vi "4Pi Test Astig.vi"(7 "Calling VI Ref":refnum<vi>) -> ()   [LabVIEW 2016]
uses:
  Hardware Configuration/Hardware Configuration Controls/Device Type.ctl
  Hardware Configuration/Hardware Configuration Controls/Device Function.ctl
  <vilib>/Utility/miscctls.llb/LVPointTypeDef.ctl
  4Pi Test Astig - Type Defs/4Pi Test Astig - Actions.ctl
  4Pi Test Astig - Type Defs/4Pi Test Astig - Notifier Type.ctl
  Device Library/Stages/Stages Controls/Stage Actions.ctl
panel:
  in  "Image Selection":i32(ring) items=["Quad 01", "Quad 02", "Quad 03", "Quad 04"]
  in  "Frame Accums.":u16=1
  in  "Start Scan":bool
  in  "Step Size (µm)":dbl=0.1
  in  "Number of Steps":u16=1
  in  "Quit":bool
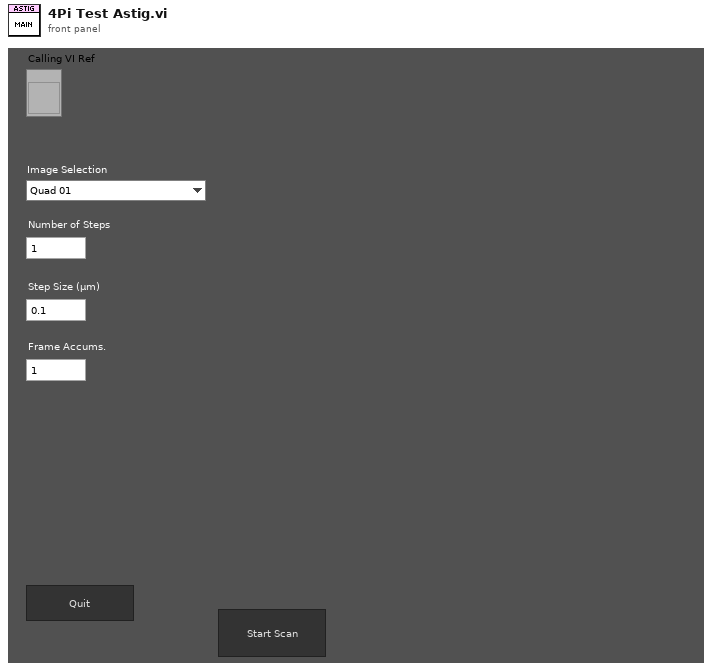
[diagram p1: front panel]
types:
  T1 = typedef "4Pi Test Astig - Actions.ctl" = enum16{"Idle", "Start Scan", "Get Image", "Move Z Stage", "Fit Astig Curves", "Quit"}
  T2 = typedef "4Pi Test Astig - Notifier Type.ctl" = cluster{"Actions":T1, "Scan Steps":u16, "Step Size (µm)":dbl, "Frame Accums":u16}
  T3 = enum16{"Always On", "Always Off", "Off While Running"}
  T4 = typedef "LVPointTypeDef.ctl" = cluster{"Horizontal":i16, "Vertical":i16}
  T5 = typedef "Device Function.ctl" = enum16{"Primary", "Secondary", "Overview", "Wide Field Drift Correction", "642 nm Excitation", "560 nm Excitation", "546 nm Excitation", "488 nm Excitation", "405 nm Excitation", "Objective Drift Correction", "Objective XY", "Objective Z", "Sample XY", "Sample Coarse Z", "Sample Z", "4Pi Lower", "4Pi Upper", "Adj Cavity"}
  T6 = typedef "Device Type.ctl" = enum16{"AOTF", "Camera", "Deformable Mirror", "Laser", "Shutter", "Stage"}
  T7 = typedef "Stage Actions.ctl" = enum16{"Get Position", "MVR", "MOVE", "HALT", "ONTARGET", "ERROR", "REFERENCE", "INIT", "VELOCITY", "STATUS", "EXIT", "HOME", "ZEROPOS", "NANOPOS", "ANALOG", "QUIT"}
  T8 = enum32{"Invalid", "Standard", "Closed", "Hidden", "Minimized", "Maximized"}
  T9 = typedef "2D Gaussian - Best Fit Parameters.ctl" = cluster{"Amplitude":dbl, "X Position":dbl, "Y Position":dbl, "X Width":dbl, "Y Width":dbl, "Offset":dbl}
  T10 = typedef "LVRectTypeDef.ctl" = cluster{"Left":i16, "Top":i16, "Right":i16, "Bottom":i16}
  T11 = typedef "LVBoundsTypeDef.ctl" = cluster{"Width":u32, "Height":u32}
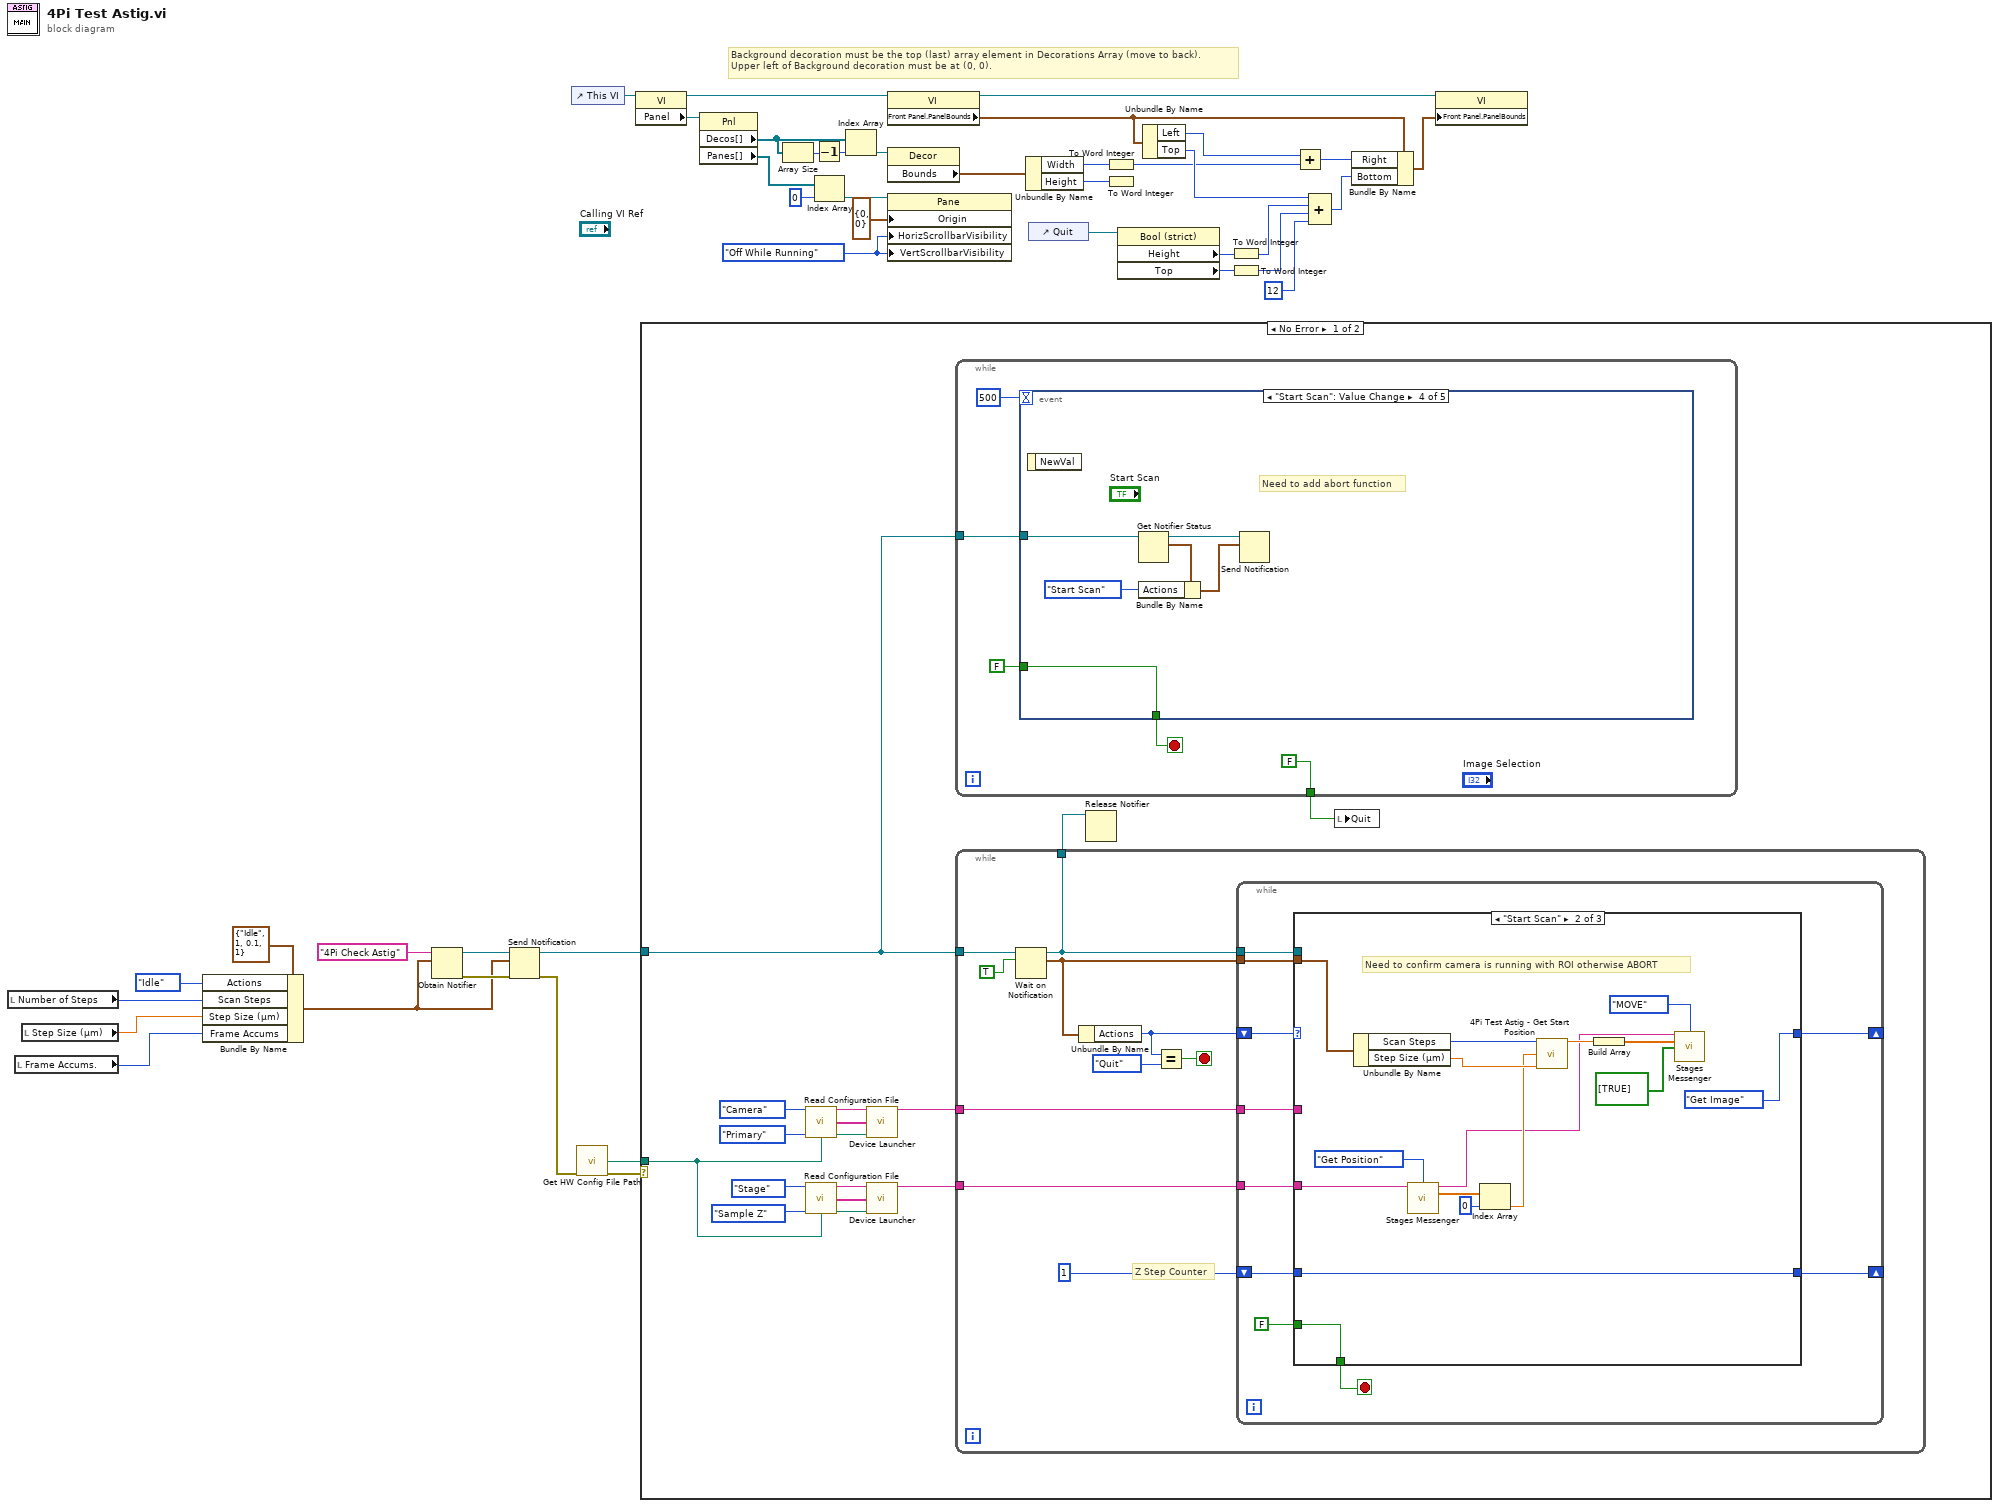
[diagram p0: block diagram]
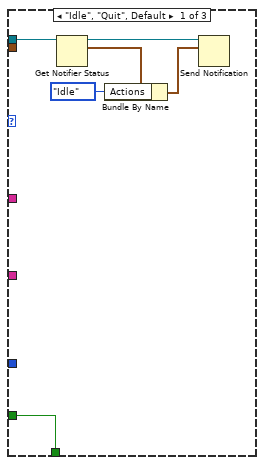
[diagram p2: hidden frame]
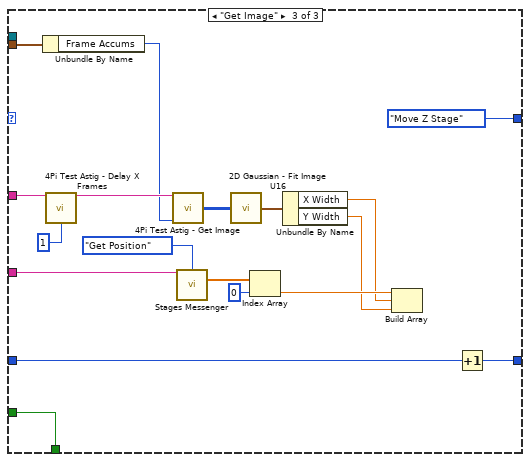
[diagram p3: hidden frame]
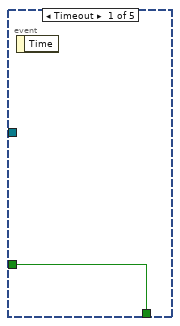
[diagram p4: hidden frame]
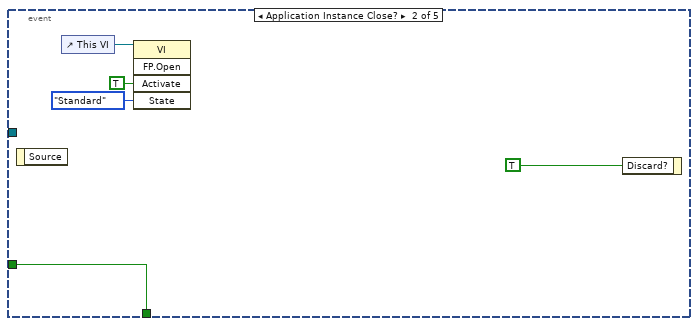
[diagram p5: hidden frame]
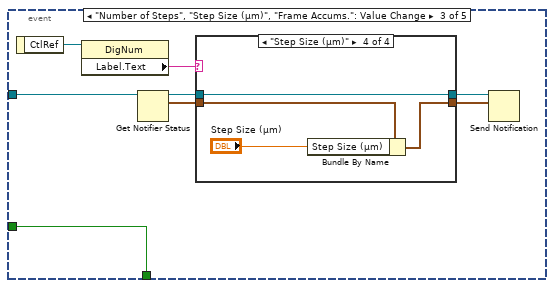
[diagram p6: hidden frame]
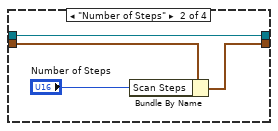
[diagram p8: hidden frame]
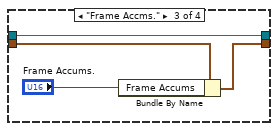
[diagram p9: hidden frame]
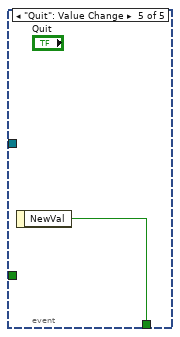
[diagram p10: hidden frame]
diagram:
  w23 = T3."Off While Running" ("Vertical Scrollbar Visibility")
  # "Background decoration must be the top (last) array element in Decorations Array (move to back).\nUpper left of Background decoration must be at (0, 0)."
  n1 = local read "Number of Steps"() -> (w3:u16)
  n2 = local read "Frame Accums."() -> (w1:u16)
  n3 = local read "Step Size (µm)"() -> (w2:dbl)
  n4 = Bundle By Name(cluster=T2 {"Actions"=enum."Idle", "Scan Steps"=1, "Step Size (µm)"=0.1, "Frame Accums"=1} ("Astig Test Data Type"), "Actions"=4Pi_Test_Astig_-_Actions."Idle", "Scan Steps"=w3, "Step Size (µm)"=w2, "Frame Accums"=w1) -> (w4:T2)
  n5 = Obtain Notifier(name (unnamed)="4Pi Check Astig", notification data type=w4) -> (notifier out=w11:refnum<notifier>, error out=w10:errorcluster)  [unwired: 2 in, 1 out]
  n6 = Send Notification(notification=w4, notifier=w11, error in (no error)=w10) -> (notifier out=w7:refnum<notifier>, error out=w8:errorcluster)
  n7 = control-ref of="This VI"() -> (w15:refnum<vi>)
  n8 = call "Get HW Config File Path.vi"("Error"=w8) -> ("File Path"=w41:path, "Error"=w42:errorcluster)  [unwired: 13 in]
  n9 = property class="VI"(reference=w15) -> (reference out=w24:refnum<vi>, "Panel"=w16:refnum<vi>)  [unwired: 1 in, 1 out]
  n10 = case shown="No Error" w42 {
    tunnel: w41 -> [w47 _]
    tunnel: w7 -> [w45 _]
    frame No Error {
      n11 = call "Read Configuration File.vi"("Device Type"=Device_Type."Camera", "Device Function"=Device_Function."Primary", "Config File Path"=w47) -> ("Unique Notifier Name"=w56:string, "Device Ports/IDs/Channels"=w58:string[], "Device Engine Path"=w57:path)  [unwired: 9 in, 1 out]
      n12 = call "Read Configuration File.vi"("Device Type"=Device_Type."Stage", "Device Function"=Device_Function."Sample Z", "Config File Path"=w47) -> ("Unique Notifier Name"=w50:string, "Device Ports/IDs/Channels"=w48:string[], "Device Engine Path"=w49:path)  [unwired: 9 in, 1 out]
      n13 = call "Device Launcher.vi"("Notifier Name"=w56, "Device Ports/IDs/Channels"=w58, "Device Engine Path"=w57) -> ("Notifier Name"=w43:string)  [unwired: 11 in, 1 out]
      n14 = call "Device Launcher.vi"("Notifier Name"=w50, "Device Ports/IDs/Channels"=w48, "Device Engine Path"=w49) -> ("Notifier Name"=w44:string)  [unwired: 11 in, 1 out]
      n15 = while {
        tunnel: [FALSE] -> w53
        tunnel: w45 -> [w119]
        stop <- w121 stop-if-true
        n16 = event shown="[3] \"Start Scan\": Value Change" {
          selector: _ -> [_ _ _ _ _]
          dyn-events: _ -> [_ _ _ _ _]
          timeout: 500 -> [_ _ _ _ _]
          tunnel: FALSE -> [w124 w128 w137 w157 _]
          tunnel: [w124 w128 w137 w157 w158] -> w121
          tunnel: w119 -> [_ _ w136 w156 _]
          event Timeout {
            n17 = event-data() -> ()  [unwired: 1 in, 1 out]
          }
          event Application Instance Close? {
            n18 = event-data() -> ()  [unwired: 1 in, 1 out]
            n19 = control-ref of="This VI"() -> (w125:refnum<vi>)
            n20 = invoke class="VI" method="FP.Open"(reference=w125, "Activate"=TRUE ("Activate?"), "State"=T8."Standard") -> ()  [unwired: 2 in, 5 out]
            n21 = event-data("Discard?"=TRUE) -> ()  [unwired: 1 in, 1 out]
          }
          event "Number of Steps", "Step Size (µm)", "Frame Accums.": Value Change {
            n22 = event-data() -> ("CtlRef"=w135:refnum<vi>)  [unwired: 1 in]
            n23 = property class="DigNum"(reference=w135) -> ("Label.Text"=w134:string)  [unwired: 1 in, 2 out]
            n24 = Get Notifier Status(notifier=w136) -> (notifier out=w133:refnum<notifier>, current notification=w132:T2)  [unwired: 1 in, 3 out]
            n25 = case shown="\"Step Size (µm)\"" w134 {
              tunnel: w133 -> [w139 w143 w147 w151]
              tunnel: w132 -> [w138 w142 w146 w150]
              tunnel: [w139 w143 w147 w151] -> w131
              tunnel: [w138 w140 w145 w149] -> w130
              frame Default {
              }
              frame "Number of Steps" {
                n26 = Bundle By Name(cluster=w142, "Scan Steps"="Number of Steps") -> (w140:T2)
              }
              frame "Frame Accms." {
                n27 = Bundle By Name(cluster=w146, "Frame Accums"="Frame Accums.") -> (w145:T2)
              }
              frame "Step Size (µm)" {
                n28 = Bundle By Name(cluster=w150, "Step Size (µm)"="Step Size (µm)") -> (w149:T2)
              }
            }
            n29 = Send Notification(notification=w130, notifier=w131) -> ()  [unwired: 1 in, 2 out]
          }
          event "Start Scan": Value Change {
            # "Need to add abort function"
            n30 = event-data() -> ()  [unwired: 1 in, 1 out]
            n31 = Get Notifier Status(notifier=w156) -> (notifier out=w155:refnum<notifier>, current notification=w154:T2)  [unwired: 1 in, 3 out]
            n32 = Bundle By Name(cluster=w154, "Actions"=4Pi_Test_Astig_-_Actions."Start Scan") -> (w153:T2)
            n33 = Send Notification(notification=w153, notifier=w155) -> ()  [unwired: 1 in, 2 out]
          }
          event "Quit": Value Change {
            n34 = event-data() -> ("NewVal"=w158:bool)  [unwired: 1 in]
          }
        }
      }
      n35 = while {
        tunnel: w45 -> [w68]
        tunnel: [w62] -> w46
        tunnel: w44 -> [w61]
        tunnel: w43 -> [w59]
        stop <- w65 stop-if-true
        # "Z Step Counter"
        n36 = Wait on Notification(notifier=w68, ignore previous (F)=TRUE) -> (notifier out=w62:refnum<notifier>, notification=w64:T2)  [unwired: 2 in, 2 out]
        n37 = Unbundle By Name(w64) -> ("Actions"=w63:T1)
        n38 = Equal?(x=w63, y=4Pi_Test_Astig_-_Actions."Quit") -> (x = y?=w65:bool)
        n39 = while {
          tunnel: w64 -> [w75]
          shift-right: [w72] -> _
          shift-left: w63 -> [w78]
          tunnel: w62 -> [w74]
          tunnel: w61 -> [w73]
          shift-right: [w70] -> _
          shift-left: 1 -> [w71]
          tunnel: w59 -> [w69]
          stop <- w76 stop-if-true
          n40 = case shown="\"Start Scan\"" w78 {
            tunnel: FALSE -> [w84 w93 w118]
            tunnel: [w84 w93 w118] -> w76
            tunnel: w75 -> [_ w100 w112]
            tunnel: w74 -> [w83 _ _]
            tunnel: w73 -> [_ w97 w106]
            tunnel: [_ 4Pi_Test_Astig_-_Actions."Get Image" ("y") 4Pi_Test_Astig_-_Actions."Move Z Stage" ("y")] -> w72
            tunnel: [_ w85 w117] -> w70
            tunnel: w71 -> [_ w85 w116]
            tunnel: w69 -> [_ _ w115]
            frame "Idle", "Quit", Default {
              n41 = Get Notifier Status(notifier=w83) -> (notifier out=w82:refnum<notifier>, current notification=w81:T2)  [unwired: 1 in, 3 out]
              n42 = Bundle By Name(cluster=w81, "Actions"=4Pi_Test_Astig_-_Actions."Idle") -> (w79:T2)
              n43 = Send Notification(notification=w79, notifier=w82) -> ()  [unwired: 1 in, 2 out]
            }
            frame "Start Scan" {
              # "Need to confirm camera is running with ROI otherwise ABORT"
              n44 = Unbundle By Name(w100) -> ("Scan Steps"=w99:u16, "Step Size (µm)"=w98:dbl)
              n45 = call "Stages Messenger.vi"("Stage Notifier Name"=w97, "Actions"=Stage_Actions."Get Position") -> ("Stage Notifier Name (Dup)"=w88:string, "Positions"=w95:dbl[])  [unwired: 10 in, 2 out]
              n46 = Index Array(array=w95, index=0) -> (element=w92:dbl)
              n47 = call "4Pi Test Astig - Get Start Position.vi"("Number of Steps"=w99, "Center Value"=w92, "Step Size"=w98) -> ("Starting Value"=w90:dbl)  [unwired: 11 in, 1 out]
              n48 = Build Array(w90) -> (w89:dbl[])
              n49 = call "Stages Messenger.vi"("Stage Notifier Name"=w88, "Actions"=Stage_Actions."MOVE", "Setpoint"=w89, "Axis"=bool[] [TRUE]) -> ()  [unwired: 8 in, 4 out]
            }
            frame "Get Image" {
              n50 = Unbundle By Name(w112) -> ("Frame Accums"=w111:u16)
              n51 = call "4Pi Test Astig - Delay X Frames.vi"("Camera Notifier Name"=w115, "Wait No. (1)"=u32 1) -> ("Camera Notifier Name (Dup)"=w113:string)  [unwired: 13 in]
              n52 = call "4Pi Test Astig - Get Image.vi"("Camera Notifier Name"=w113, "Frame Accums."=w111) -> ("Image Out"=w110:u16[][])  [unwired: 13 in]
              n53 = call "Stages Messenger.vi"("Stage Notifier Name"=w106, "Actions"=Stage_Actions."Get Position") -> ("Positions"=w108:dbl[])  [unwired: 10 in, 3 out]
              n54 = call "2D Gaussian - Fit Image U16.vi"("Image In (U16)"=w110) -> ("Best Fit Params"=w104:T9)  [unwired: 14 in]
              n55 = Index Array(array=w108, index=0) -> (element=w105:dbl)
              n56 = Unbundle By Name(w104) -> ("X Width"=w102:dbl, "Y Width"=w103:dbl)
              n57 = Build Array(w105, w102, w103) -> ()  [unwired: 1 out]
              n58 = Increment(x=w116) -> (x+1=w117:i32)
            }
          }
        }
      }
      n59 = Release Notifier(notifier=w46) -> ()  [unwired: 2 in, 3 out]
      n60 = local write "Quit"(w53) -> ()
    }
    frame Error {
    }
  }
  n61 = property class="Pnl"(reference=w16) -> ("Decos[]"=w14:refnum<vi>[], "Panes[]"=w20:refnum<vi>[])  [unwired: 1 in, 2 out]
  n62 = Array Size(array=w14) -> (size(s)=w12:i32)
  n63 = Decrement(x=w12) -> (x-1=w13:i32)
  n64 = Index Array(array=w20, index=0) -> (element=w19:refnum<vi>)
  n65 = Index Array(array=w14, index=w13) -> (element=w22:refnum<vi>)
  n66 = property class="VI"(reference=w24) -> (reference out=w26:refnum<vi>, "Front Panel.PanelBounds"=w27:T10)  [unwired: 1 in, 1 out]
  n67 = property class="Decor"(reference=w22) -> ("Bounds"=w25:T11)  [unwired: 1 in, 2 out]
  n68 = property class="Pane"(reference=w19, "Origin"=T4 {"Horizontal"=0, "Vertical"=0}, "HorizScrollbarVisibility"=w23, "VertScrollbarVisibility"=w23) -> ()  [unwired: 1 in, 2 out]
  n69 = Unbundle By Name(w25) -> ("Width"=w30:u32, "Height"=w33:u32)
  n70 = control-ref of="Quit"() -> (w17:refnum<vi>)
  n71 = To Word Integer(number=w30) -> (16bit integer=w32:i16)
  n72 = To Word Integer(number=w33) -> ()  [unwired: 1 out]
  n73 = property class="Bool (strict)"(reference=w17) -> ("Height"=w35:u32, "Top"=w36:i32)  [unwired: 1 in, 2 out]
  n74 = Unbundle By Name(w27) -> ("Left"=w29:i16, "Top"=w40:i16)
  n75 = To Word Integer(number=w35) -> (16bit integer=w38:i16)
  n76 = To Word Integer(number=w36) -> (16bit integer=w39:i16)
  n77 = Add(x=w29, y=w32) -> (x+y=w31:i16)
  n78 = Compound Arithmetic op=ADD(w40, w38, w39, i16 12 ("y")) -> (w34:i16)
  n79 = Bundle By Name(cluster=w27, "Right"=w31, "Bottom"=w34) -> (w28:T10)
  n80 = property class="VI"(reference=w26, "Front Panel.PanelBounds"=w28) -> ()  [unwired: 1 in, 2 out]
